vi "While_loop.vi"() -> ()   [LabVIEW 2017]
panel:
  out "Numeric":dbl
  in  "stop":bool
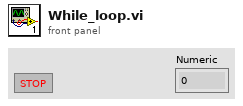
[diagram p1: front panel]
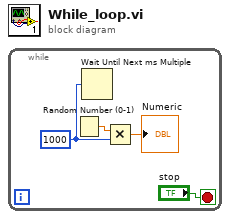
[diagram p0: block diagram]
diagram:
  n1 = while {
    stop <- "stop" stop-if-true
    w1 = 1000
    n2 = Random Number (0-1)() -> (number: 0 to 1=w3:dbl)
    n3 = Wait Until Next ms Multiple(millisecond multiple=w1) -> ()  [unwired: 1 out]
    n4 = Multiply(x=w3, y=w1) -> (x*y=→"Numeric":dbl)
  }
